vi "Update_Simon_Scores.vi"(9 "Score":i32, 10 "Position":i32, 11 "LoopLength":i32) -> (1 "New Score":i32, 2 "Next Pos":i32, 3 "Case Selector out":T1(ring))   [LabVIEW 2015]
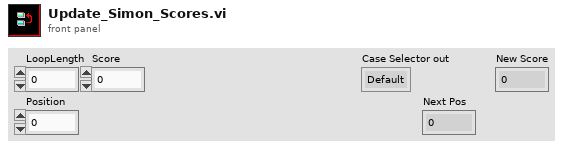
[diagram p1: front panel]
types:
  T1 = enum16{"Default", "Initialization", "New Random", "Display", "Player Choice", "IsCorrect", "Loss", "Error_Case", "Instructions"}
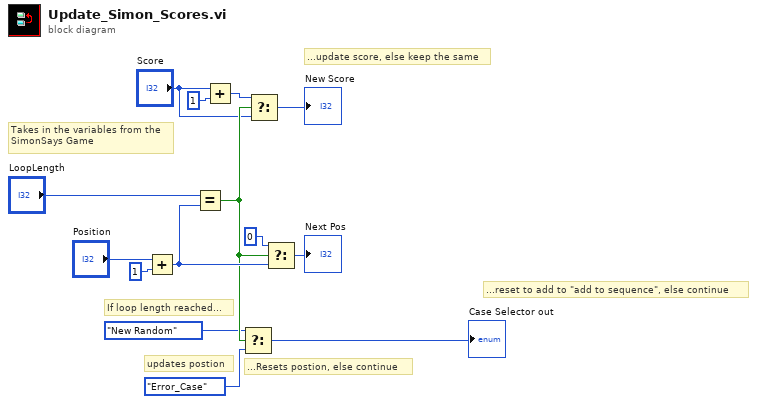
[diagram p0: block diagram]
diagram:
  # "If loop length reached..."
  # "...update score, else keep the same"
  # "...reset to add to \"add to sequence\", else continue"
  # "...Resets postion, else continue"
  # "updates postion"
  # "Takes in the variables from the\nSimonSays Game"
  n1 = Add(x="Position", y=1) -> (x+y=w12:i32)
  n2 = Equal?(x="LoopLength", y=w12) -> (x = y?=w9:bool)
  n3 = Add(x="Score", y=1) -> (x+y=w10:i32)
  n4 = Select(t=T1."New Random", s=w9, f=T1."Error_Case") -> (s? t:f=→"Case Selector out":T1)
  n5 = Select(t=w10, s=w9, f="Score") -> (s? t:f=→"New Score":i32)
  n6 = Select(t=0 ("f"), s=w9, f=w12) -> (s? t:f=→"Next Pos":i32)
